vi "Transfer Compressed Data (SubVI).vi"(11 "Read":bool) -> (0 "Data Valid":bool, 3 "Data Out":u64)   [LabVIEW 2014]
uses:
  Controls (FPGA)/Send Display Data.ctl
  <vilib>/rvi/Emulation/niFpgaEmulationIsFPGAContextNoSignature.vi
  <vilib>/rvi/Emulation/niFpgaSctlEmulationGetInTimedLoop.vi
  <vilib>/rvi/errors/niFpgaSetErrorForExecOnDevCompSimple.vi
  <vilib>/rvi/eio/common/nirviEmuReportErrorAndStop.vi
  <vilib>/rvi/DataTransferAndStorage/Container/Common/niFpgaContainerGetUniqueNameForEmu.vi
  <vilib>/rvi/FIFO/Fifo_Resource/nirvififoEmulationSetSize.vi
  <vilib>/rvi/FIFO/Fifo_Resource/nirviFifoEmulationQueueMgr.vi
  <instcachedir>/0/nirviFifoEmulationQueueMgr_E5CAEC123FF24DC58D834DCA3CDAA9B5.lvgen/nirviFifoEmulationQueueMgr_E5CAEC123FF24DC58D834DCA3CDAA9B5_007.vi
  <vilib>/Utility/error.llb/Clear Errors.vi
  <vilib>/rvi/FIFO/Fifo_Resource/nirvififoEmulationCreateLock.vi
  <vilib>/rvi/Emulation/niFpgaProcessEmulError.vi
  <vilib>/rvi/FIFO/Fifo_Resource/nirvififoEmulationObtainLock.vi
  <vilib>/rvi/FIFO/Fifo_Resource/nirvififoEmulationReleaseLock.vi
  <vilib>/rvi/occurrence/nirviWaitOnOccurrenceBase.vi
  <vilib>/rvi/errors/nirviReportUnexpectedCaseInternalError.vi
  <vilib>/rvi/errors/nirviReportUnexpectedCaseInternalError (U32).vi
  <vilib>/rvi/DataTransferAndStorage/Container/XNode/niFpgaContainer.xnode
  <vilib>/rvi/FIFO/Fifo_Resource/nirvififoEmulationRead.vi
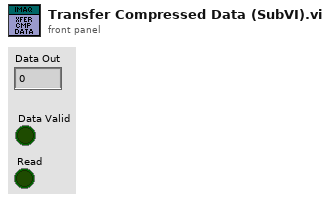
[diagram p1: front panel]
types:
  T1 = typedef "Send Display Data.ctl" = enum16{"Wait", "Pass N Clock Cycles", "Send Data Lower 64", "Send Data Upper 64"}
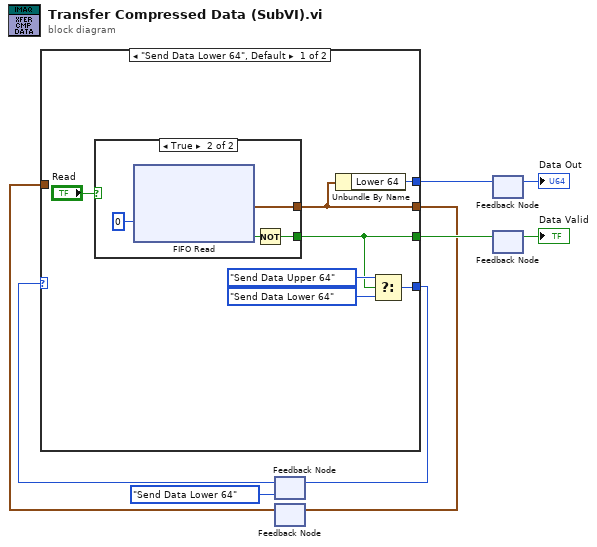
[diagram p0: block diagram]
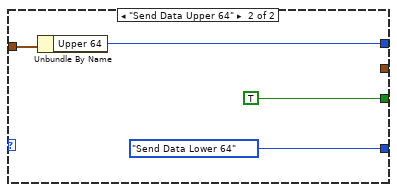
[diagram p3: hidden frame]
diagram:
  n1 = feedback #1(Send_Display_Data."Send Data Lower 64" ("f")) -> (w4:T1)
  n2 = feedback #2() -> (w7:cluster{"Lower 64":u64, "Upper 64":u64})  [unwired: 1 in]
  n3 = case shown="\"Send Data Lower 64\", Default" w4 {
    tunnel: [w15 Send_Display_Data."Send Data Lower 64" ("f")] -> w3
    tunnel: [w13 _] -> w6
    tunnel: [w14 TRUE] -> w9
    tunnel: w7 -> [_ w24]
    tunnel: [w12 w23] -> w8
    frame "Send Data Lower 64", Default {
      n4 = case shown="True" "Read" {
        tunnel: [_ w18] -> w14
        tunnel: [_ w17] -> w13
        frame False {
        }
        frame True {
          n5 = xnode ("FIFO Read")("Timeout"=0) -> ("Element"=w17:cluster{"Lower 64":u64, "Upper 64":u64}, "Timed Out?"=w19:bool)  [unwired: 1 in, 1 out]
          n6 = Not(x=w19) -> (.not. x?=w18:bool)
        }
      }
      n7 = Unbundle By Name(w13) -> ("Lower 64"=w12:u64)
      n8 = Select(t=Send_Display_Data."Send Data Upper 64" ("f"), s=w14, f=Send_Display_Data."Send Data Lower 64") -> (s? t:f=w15:T1)
    }
    frame "Send Data Upper 64" {
      n9 = Unbundle By Name(w24) -> ("Upper 64"=w23:u64)
    }
  }
  n10 = feedback-in #1(w3) -> ()
  n11 = feedback-in #2(w6) -> ()
  n12 = feedback-in #3(w8) -> ()
  n13 = feedback #3() -> (→"Data Out":u64)  [unwired: 1 in]
  n14 = feedback-in #4(w9) -> ()
  n15 = feedback #4() -> (→"Data Valid":bool)  [unwired: 1 in]
